vi "Run.vi"(8 "error in (no error)":errorcluster, 11 "C37.118 PMU in":refnum<class "C37.118 PMU.lvclass">) -> (0 "error out":errorcluster, 1 "DataValid":bool, 2 "clSensorData":T1, 3 "C37.118 PMU out":refnum<class "C37.118 PMU.lvclass">)   [LabVIEW 2018, in "SensorPlugins.lvlib" / "C37.118 PMU.lvclass"]
uses:
  C37.118 PMU.lvclass
  SensorShared/clSensorData.ctl
  C37.118 PMU.lvclass/C37.118 PMU.ctl
  Accessors/Read DataSocket.vi
  <userlib>/NIST/Socket Class/Classes/Socket.Base/Socket.Base.lvclass
  SensorShared/SensorShared.lvlib
  PmuBaseClass/PmuBase.lvclass
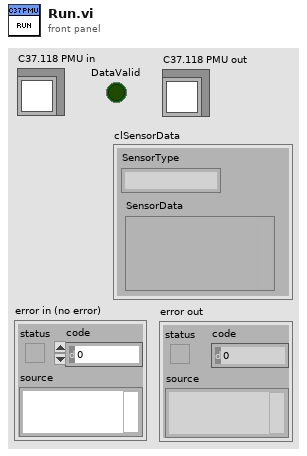
[diagram p1: front panel]
types:
  T1 = typedef "SensorShared.lvlib/clSensorData.ctl" = cluster{"SensorType":string, "SensorData":variant}
  T2 = typedef "SensorPlugins.lvlib/PmuBase.lvclass/PMUDataType.ctl" = enum16{"undefined", "data", "header", "config 1", "config 2", "config 3", "command"}
  T3 = typedef "SensorPlugins.lvlib/PmuBase.lvclass/PmuData.ctl" = cluster{"Timestamp":dbl, "Synx":cdb[], "Freq":dbl, "ROCOF":dbl, "ID":i16}
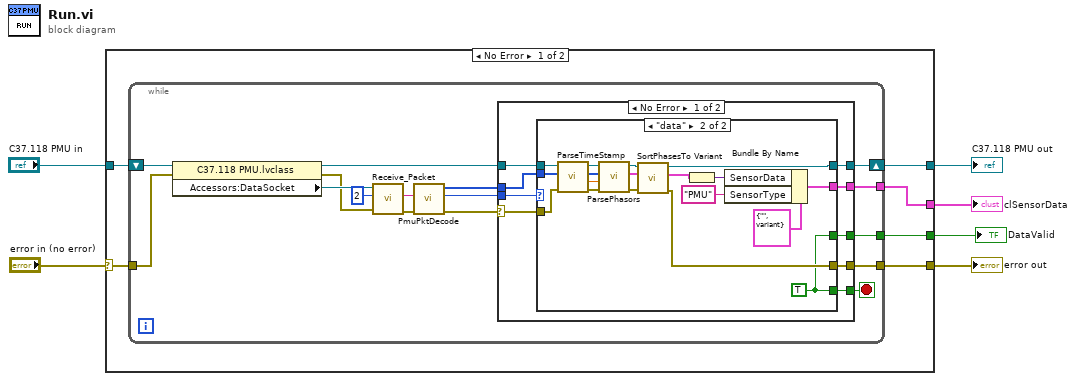
[diagram p0: block diagram]
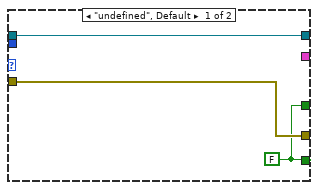
[diagram p2: hidden frame]
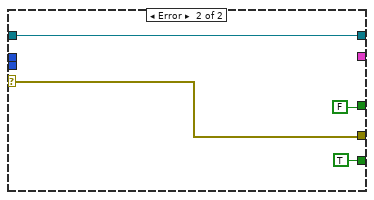
[diagram p3: hidden frame]
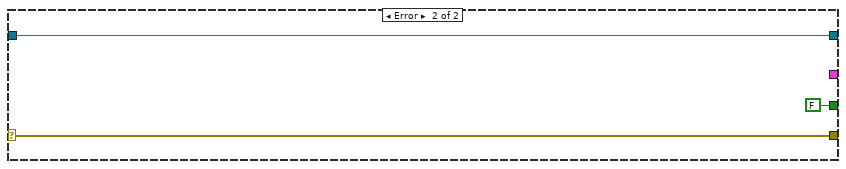
[diagram p4: hidden frame]
diagram:
  n1 = case shown="No Error" "error in (no error)" {
    selector: "error in (no error)" -> [w11 w65]
    tunnel: [w9 w65] -> w5
    tunnel: "C37.118 PMU in" -> [w12 w64]
    tunnel: [w10 w64] -> w3
    tunnel: [w8 _] -> w2
    tunnel: [w7 FALSE] -> w1
    frame No Error {
      n2 = while {
        tunnel: w11 -> [w25]
        shift-right: [w20] -> w10
        shift-left: w12 -> [w28]
        tunnel: [w16] -> w9
        tunnel: [w15] -> w8
        tunnel: [w13] -> w7
        stop <- w17 stop-if-true
        n3 = property class="C37.118 PMU.lvclass"(reference=w28, error in=w25) -> (reference out=w21:refnum<class "C37.118 PMU.lvclass">, error out=w26:errorcluster, "Accessors:DataSocket"=w27:refnum<class "Socket.Base.lvclass">)
        n4 = call-dynamic "Receive_Packet.vi"("error in (no error)"=w26, "bufsize (0)"=u32 2, "Socket.Base in"=w27) -> ("error out"=w23:errorcluster, "data_out"=w22:string)  [unwired: 5 in, 2 out]
        n5 = call "PmuPktDecode.vi"("error in (no error)"=w23, "PktData"=w22) -> ("error out"=w14:errorcluster, "PMUDataType"=w18:T2, "PktData"=w19:u8[])  [unwired: 5 in, 2 out]
        n6 = case shown="No Error" w14 {
          selector: w14 -> [w30 w60]
          tunnel: w21 -> [w37 w61]
          tunnel: [w36 w61] -> w20
          tunnel: w19 -> [w35 _]
          tunnel: w18 -> [w34 _]
          tunnel: [w33 TRUE] -> w17
          tunnel: [w32 w60] -> w16
          tunnel: [w31 _] -> w15
          tunnel: [w29 FALSE] -> w13
          frame No Error {
            n7 = case shown="\"data\"" w34 {
              tunnel: w37 -> [w40 w58]
              tunnel: [w40 w43] -> w36
              tunnel: w35 -> [_ w57]
              tunnel: [w38 w41] -> w33
              tunnel: w30 -> [w39 w56]
              tunnel: [w39 w44] -> w32
              tunnel: [_ w48] -> w31
              tunnel: [w38 w41] -> w29
              frame "undefined", Default {
                w38 = FALSE
              }
              frame "data" {
                w41 = TRUE
                n8 = call "ParseTimeStamp.vi"("error in (no error)"=w56, "PktData"=w57, "C37.118 PMU in"=w58) -> ("error out"=w55:errorcluster, "Seconds"=w52:ext, "PktData"=w53:u8[], "C37.118 PMU out"=w54:refnum<class "C37.118 PMU.lvclass">)  [unwired: 2 in, 3 out]
                n9 = call "ParsePhasors.vi"("error in (no error)"=w55, "TimeStamp"=w52, "PktData"=w53, "C37.118 PMU in"=w54) -> ("error out"=w47:errorcluster, "PmuReport"=w46:T3, "C37.118 PMU out"=w45:refnum<class "C37.118 PMU.lvclass">)  [unwired: 5 in]
                n10 = call "SortPhases.vi"("error in (no error)"=w47, "PmuReport"=w46, "C37.118 PMU in"=w45) -> ("error out"=w44:errorcluster, "PmuReport 2"=w42:T3, "C37.118 PMU out"=w43:refnum<class "C37.118 PMU.lvclass">)  [unwired: 6 in]
                n11 = To Variant(anything=w42) -> (Variant=w50:variant)
                n12 = Bundle By Name(cluster=T1 {"SensorType"="", "SensorData"=variant} ("clSensorData"), "SensorData"=w50, "SensorType"="PMU") -> (w48:T1)
              }
            }
          }
          frame Error {
          }
        }
      }
    }
    frame Error {
    }
  }
  "error out" <- w5
  "C37.118 PMU out" <- w3
  "clSensorData" <- w2
  "DataValid" <- w1
